vi "AlazarBeforeAsyncRead.vi"(0 "Handle":u64, 1 "Channel Select":u32(ring)=1 items=["A"=1, "B"=2, "A + B"=3, "C"=4, "A + C"=5, "A + B"=6, "D"=8, "A + D"=9, "B + D"=10, "C + D"=12, "A + B + C + D"=15], 2 "Transfer Offset":u32, 3 "Transfer Length":u32, 4 "Records Per Buffer":u32, 5 "Records Per Acquisition":u32, 6 "Flags":u32, 7 "error in (no error)":errorcluster) -> (20 "Handle":u64, 26 "Return Code":u32, 27 "error out":errorcluster)   [LabVIEW 2018]
doc: "Configure a board to make an asynchronous AutoDMA acquisition."
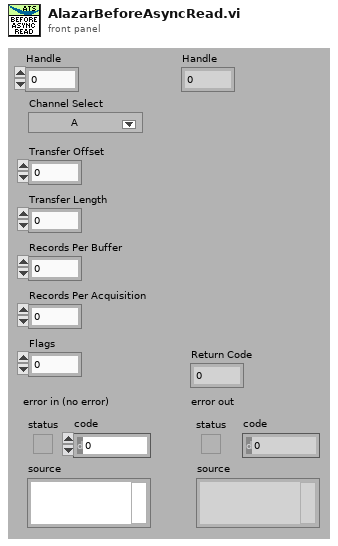
[diagram p1: front panel]
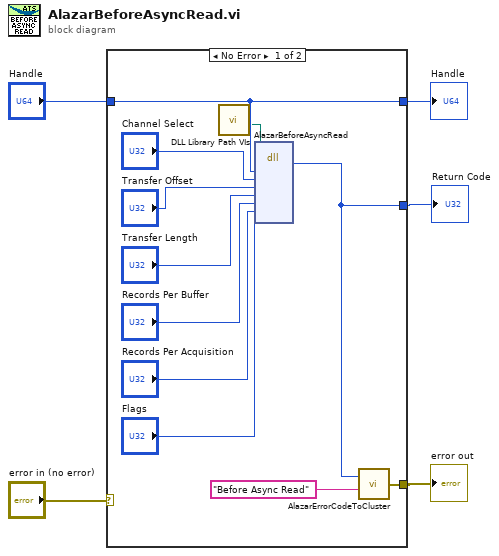
[diagram p0: block diagram]
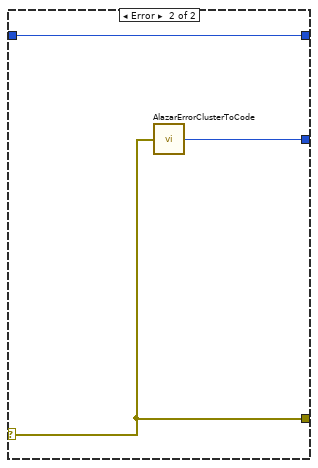
[diagram p2: hidden frame]
diagram:
  n1 = case shown="No Error" "error in (no error)" {
    selector: "error in (no error)" -> [_ w19]
    tunnel: [w14 w19] -> w4
    tunnel: [w16 w18] -> w3
    tunnel: "Handle" -> [w13 w17]
    tunnel: [w13 w17] -> w1
    frame No Error {
      n2 = call "DLL Library Path VIs.vi"() -> ("Alazar"=w6:path)  [unwired: 5 in, 6 out]
      n3 = dll-call lib="C:/Project/SerialSectOCT - FFT GPU/SerialSectOCT/Labview Software/DLL/ATSApi.dll" fn="AlazarBeforeAsyncRead"(path in=w6, "handle"=w13, "channelSelect"="Channel Select", "transferOffset"="Transfer Offset", "transferLength"="Transfer Length", "recordsPerBuffer"="Records Per Buffer", "recordsCount"="Records Per Acquisition", "cFlags"="Flags") -> ("return type"=w16:u32)  [unwired: 9 in, 2 out]
      n4 = call "AlazarErrorCodeToCluster.vi"("Message"="Before Async Read", "Error Code"=w16) -> ("error out"=w14:errorcluster)
    }
    frame Error {
      n5 = call "AlazarErrorClusterToCode.vi"("error in (no error)"=w19) -> ("Error Code"=w18:u32)
    }
  }
  "Handle" <- w1
  "error out" <- w4
  "Return Code" <- w3
